vi "BLDC Encoder.vi"(2 "Encoder Reset Value":i32, 5 "Encoder Reset":bool, 6 "A":refnum<k21>, 8 "B":refnum<k21>, 10 "C":refnum<k21>) -> (14 "Encoder RAW A/B/C":fxp<+,3,3> format="%02b", 17 "Encoder Counter":i32, 19 "BLDC State":T1(ring))   [LabVIEW 2019]
uses:
  <vilib>/rvi/eio/common/nirviEmuTemplateMethod_errors.vi
  <vilib>/eio/EIONode/EIONode.xnode
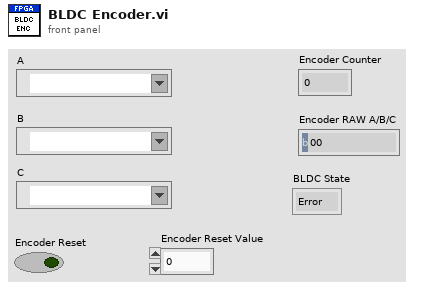
[diagram p1: front panel]
types:
  T1 = enum16{"Error", "Step 1", "Step 2", "Step 3", "Step 4", "Step 5", "Step 6"}
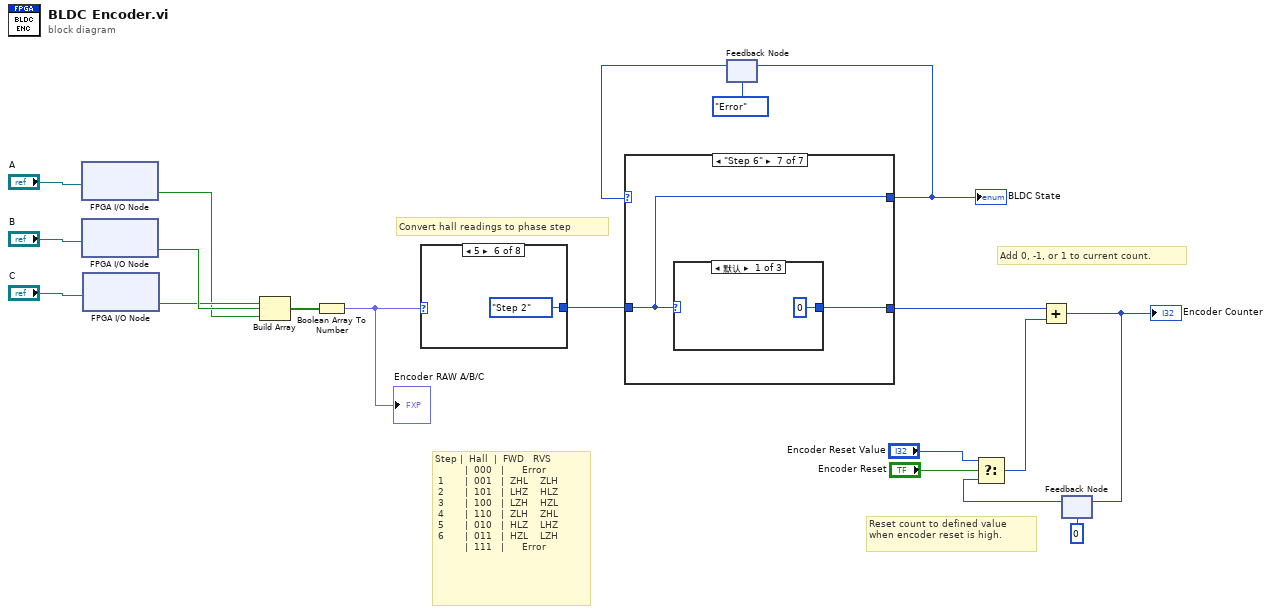
[diagram p0: block diagram]
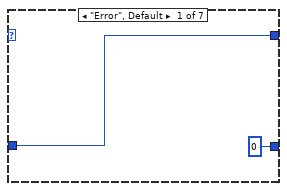
[diagram p2: hidden frame]
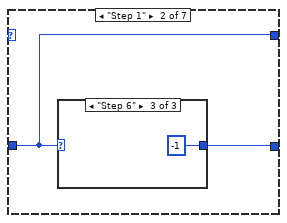
[diagram p3: hidden frame]
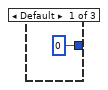
[diagram p4: hidden frame]
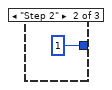
[diagram p5: hidden frame]
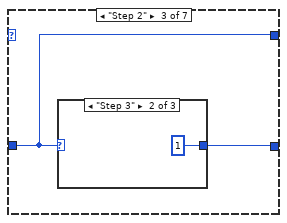
[diagram p6: hidden frame]
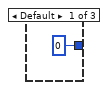
[diagram p7: hidden frame]
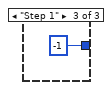
[diagram p8: hidden frame]
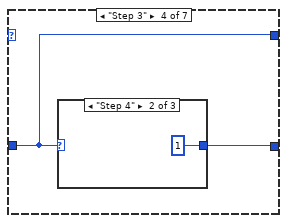
[diagram p9: hidden frame]
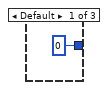
[diagram p10: hidden frame]
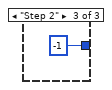
[diagram p11: hidden frame]
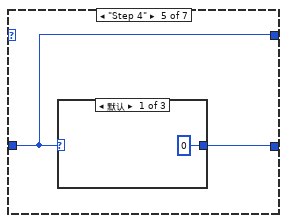
[diagram p12: hidden frame]
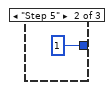
[diagram p13: hidden frame]
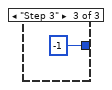
[diagram p14: hidden frame]
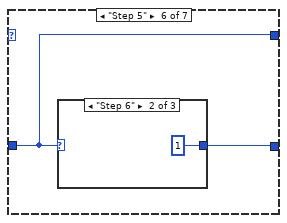
[diagram p15: hidden frame]
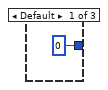
[diagram p16: hidden frame]
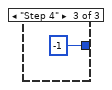
[diagram p17: hidden frame]
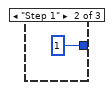
[diagram p18: hidden frame]
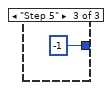
[diagram p19: hidden frame]
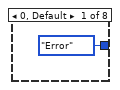
[diagram p20: hidden frame]
diagram:
  # "Step |  Hall  |  FWD   RVS\n          |  000   |      Error\n 1       |  001   |  ZHL    ZLH\n 2       |  101   |  LHZ    HLZ\n 3       |  100   |  LZH    HZL\n 4       |  110   |  ZLH    ZHL\n 5       |  010   |  HLZ    LHZ\n 6       |  011   |  HZL    LZH\n          |  111   |      Error"
  # "Convert hall readings to phase step"
  # "Reset count to defined value\nwhen encoder reset is high."
  # "Add 0, -1, or 1 to current count."
  n1 = xnode "FPGA I/O Node"("FPGA I/O输入"="A") -> ("I/O项"=w1:bool)  [unwired: 1 out]
  n2 = xnode "FPGA I/O Node"("FPGA I/O输入"="B") -> ("I/O项"=w16:bool)  [unwired: 1 out]
  n3 = xnode "FPGA I/O Node"("FPGA I/O输入"="C") -> ("I/O项"=w2:bool)  [unwired: 1 out]
  n4 = Build Array(w2, w16, w1) -> (w19:bool[])
  n5 = Boolean Array To Number(Boolean array=w19) -> (number=w8:fxp<+,3,3>)
  "Encoder RAW A/B/C" <- w8
  n6 = case shown="5" w8 {
    tunnel: [T1."Error" T1."Step 1" T1."Step 5" T1."Step 6" T1."Step 3" T1."Step 2" T1."Step 4" T1."Error"] -> w4
    frame 0, Default {
    }
    frame 1 {
    }
    frame 2 {
    }
    frame 3 {
    }
    frame 4 {
    }
    frame 5 {
    }
    frame 6 {
    }
    frame 7 {
    }
  }
  n7 = feedback #1(T1."Error") -> (w6:T1)
  n8 = case shown="\"Step 6\"" w6 {
    tunnel: [w28 w30 w35 w40 w45 w50 w55] -> w7
    tunnel: [0 w31 w36 w41 w46 w51 w56] -> w3
    tunnel: w4 -> [w28 w30 w35 w40 w45 w50 w55]
    frame "Error", Default {
    }
    frame "Step 1" {
      n9 = case shown="\"Step 6\"" w30 {
        tunnel: [0 1 -1] -> w31
        frame Default {
        }
        frame "Step 2" {
        }
        frame "Step 6" {
        }
      }
    }
    frame "Step 2" {
      n10 = case shown="\"Step 3\"" w35 {
        tunnel: [0 1 -1] -> w36
        frame Default {
        }
        frame "Step 3" {
        }
        frame "Step 1" {
        }
      }
    }
    frame "Step 3" {
      n11 = case shown="\"Step 4\"" w40 {
        tunnel: [0 1 -1] -> w41
        frame Default {
        }
        frame "Step 4" {
        }
        frame "Step 2" {
        }
      }
    }
    frame "Step 4" {
      n12 = case shown="默认" w45 {
        tunnel: [0 1 -1] -> w46
        frame Default {
        }
        frame "Step 5" {
        }
        frame "Step 3" {
        }
      }
    }
    frame "Step 5" {
      n13 = case shown="\"Step 6\"" w50 {
        tunnel: [0 1 -1] -> w51
        frame Default {
        }
        frame "Step 6" {
        }
        frame "Step 4" {
        }
      }
    }
    frame "Step 6" {
      n14 = case shown="默认" w55 {
        tunnel: [0 1 -1] -> w56
        frame Default {
        }
        frame "Step 1" {
        }
        frame "Step 5" {
        }
      }
    }
  }
  "BLDC State" <- w7
  n15 = feedback-in #1(w7) -> ()
  n16 = feedback #2(0) -> (w13:i32)
  n17 = Select(t="Encoder Reset Value", s="Encoder Reset", f=w13) -> (s? t:f=w11:i32)
  n18 = Add(x=w3, y=w11) -> (x+y=w15:i32)
  "Encoder Counter" <- w15
  n19 = feedback-in #2(w15) -> ()
